vi "CC Script Parse Focus Absolute.vi"(8 "error in (no error)":errorcluster, 9 "To Script?":bool, 10 "Move parm in":T1, 11 "FocusMoveAbsolute Parameters":string="Wheel1=3,Wheel2=5") -> (0 "error out":errorcluster, 2 "Script Out":string="ObjectName \"RA\":\"123.456\",\"DEC\":\"4546.54\"", 3 "Filter Wheel parameters in":T1)   [LabVIEW 2024]
uses:
  Focus/Focus cluster MoveFocus Command Parameters.ctl
  <vilib>/regexp/Match Regular Expression.xnode
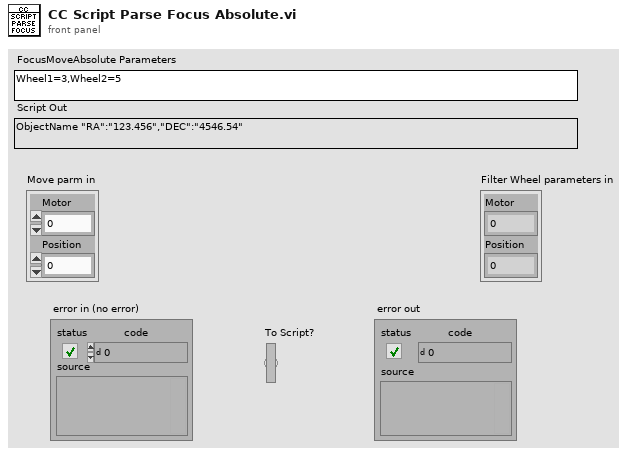
[diagram p1: front panel]
types:
  T1 = typedef "Focus cluster MoveFocus Command Parameters.ctl" = cluster{"Motor":i32, "Position":i32}
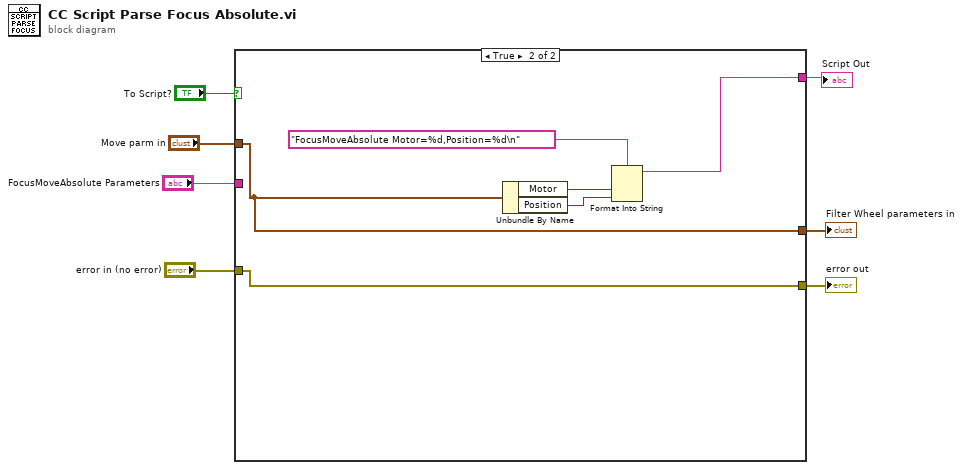
[diagram p0: block diagram]
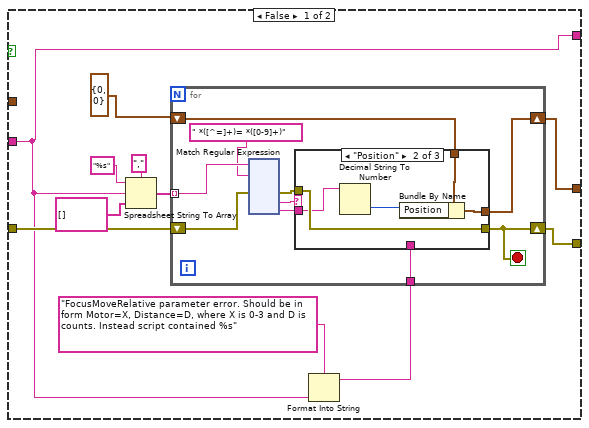
[diagram p2: hidden frame]
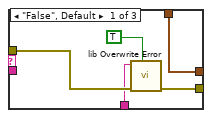
[diagram p3: hidden frame]
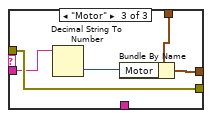
[diagram p4: hidden frame]
diagram:
  n1 = case shown="True" "To Script?" {
    tunnel: [w18 w166] -> w7
    tunnel: "error in (no error)" -> [w17 w164]
    tunnel: [w9 w164] -> w5
    tunnel: "FocusMoveAbsolute Parameters" -> [w12 _]
    tunnel: "Move parm in" -> [_ w166]
    tunnel: [w12 w165] -> w2
    frame False {
      n2 = Spreadsheet String To Array(delimiter (Tab)=",", format string="%s", spreadsheet string=w12, array type (2D Dbl)=string[] []) -> (array=w11:string[])
      n3 = Format Into String(format string="FocusMoveRelative parameter error. Should be in form Motor=X, Distance=D, where X is 0-3 and D is counts. Instead script contained %s", w12) -> (resulting string=w10:string)  [unwired: 2 in, 1 out]
      n4 = for {
        shift-right: [w27] -> w18
        shift-left: T1 {"Motor"=0, "Position"=0} ("Move parm in") -> [w28]
        tunnel: w11 -> [w26] mode=indexing
        tunnel: w10 -> [w20]
        shift-right: [w19] -> w9
        shift-left: w17 -> [w22]
        stop <- w19 stop-if-true
        n5 = xnode "Match Regular Expression"("input string"=w26, "regular expression"=" *([^=]+)= *([0-9]+)" ("format string"), "error in"=w22) -> ("error out"=w21:errorcluster, "submatch 1"=w24:string, "submatch 2"=w23:string)  [unwired: 3 in, 4 out]
        n6 = case shown="\"Position\"" w24 {
          tunnel: w28 -> [w30 w38 w43]
          tunnel: [w30 w37 w42] -> w27
          tunnel: w23 -> [_ w35 w40]
          tunnel: w21 -> [w33 w36 w41]
          tunnel: w20 -> [w32 _ _]
          tunnel: [w31 w36 w41] -> w19
          frame "False", Default {
            n7 = call "lib Overwrite Error.vi"("Force Error?"=TRUE, "error in (no error)"=w33, "Error Message"=w32) -> ("error out"=w31:errorcluster)  [unwired: 8 in]
          }
          frame "Position" {
            n8 = Decimal String To Number(string=w35) -> (number=w34:i32)  [unwired: 2 in, 1 out]
            n9 = Bundle By Name(cluster=w38, "Position"=w34) -> (w37:T1)
          }
          frame "Motor" {
            n10 = Decimal String To Number(string=w40) -> (number=w39:i32)  [unwired: 2 in, 1 out]
            n11 = Bundle By Name(cluster=w43, "Motor"=w39) -> (w42:T1)
          }
        }
      }
    }
    frame True {
      n12 = Unbundle By Name(w166) -> ("Motor"=w168:i32, "Position"=w167:i32)
      n13 = Format Into String(format string="FocusMoveAbsolute Motor=%d,Position=%d\n", w168, w167) -> (resulting string=w165:string)  [unwired: 2 in, 1 out]
    }
  }
  "error out" <- w5
  "Filter Wheel parameters in" <- w7
  "Script Out" <- w2
